vi "PV MiniTest Current State.vi"(8 "error in (no error)":errorcluster, 10 "Adress of unit":u16=1 min=1 max=999 step=1, 11 "VISA session":refnum<visa-resource-name>) -> (0 "error out":errorcluster, 1 "State out":u8(ring) items=["Power on"=0, "Power on (wait)"=2, "Wait HV-off stable"=3, "Wait HV-on stable"=4, "Ignition optimization"=5, "Wait for ignition"=6, "Wait for current"=7, "Wait for stable"=8, "Wait for vacuum"=10, "Heating"=20, "Measure"=30, "Error (new)"=100, "Error"=102, "Unrecoverable error (new)"=104, "Unrecoverable error"=106, "SW update"=110], 2 "response (data) out":string, 3 "dup VISA session":refnum<visa-resource-name>)   [LabVIEW 2021, in "Pfeiffer Vacuum.lvlib"]
doc: "This VI allows you to take simple \"Current State (Para 666)\" measurements from the MiniTest."
uses:
  <instrlib>/Pfeiffer Vacuum/Pfeiffer Vacuum.lvlib
panel:
  # "Current State (read only)"
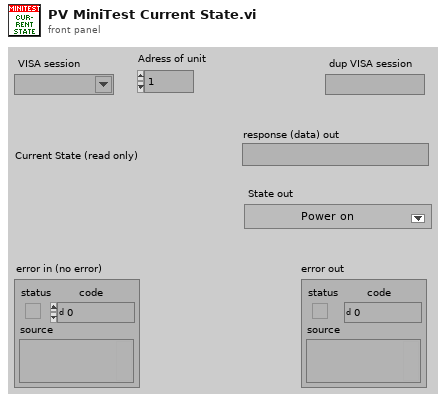
[diagram p1: front panel]
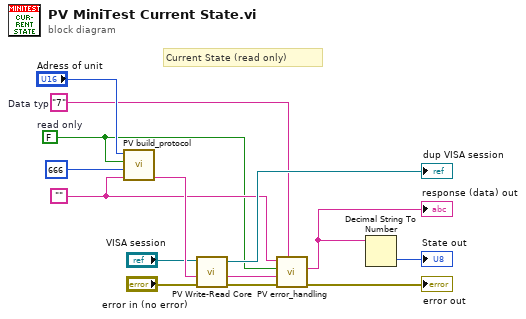
[diagram p0: block diagram]
diagram:
  w8 = "7"  # Data typ
  w9 = ""
  w7 = FALSE  # read only
  # "Current State (read only)"
  n1 = call <instrlib>:"PV build_protocol.vi"("Data"=w9, "Parameter-number"=u16 666, "parameter\nread<->describe"=w7, "Adress"="Adress of unit") -> ("output"=w12:string)  [unwired: 3 in]
  n2 = call <instrlib>:"PV Write-Read Core.vi"("error in"="error in (no error)", "Write data in"=w12, "VISA session"="VISA session") -> ("error out"=w11:errorcluster, "response (data) out"=w3:string, "dup VISA session"=→"dup VISA session":refnum<visa-resource-name>)  [unwired: 2 in]
  n3 = call <instrlib>:"PV error_handling.vi"("Data Typ in"=w8, "error in"=w11, "response (data) in"=w3, "Parameter\nread only<->describe"=w7, "data in"=w9) -> ("error out"=→"error out":errorcluster, "Data out"=w2:string)  [unwired: 4 in, 1 out]
  "response (data) out" <- w2
  n4 = Decimal String To Number(string=w2) -> (number=→"State out":i32)  [unwired: 2 in, 1 out]
